vi "Translator System API.vi"(0 "Input":variant=variant("Function Name"=variant(string "Strip Path"), "Input Datatypes"=variant(string[] ["error", "int"]), "Inputs"=variant(string[] ["error in", "x"]), "Node refnum"=variant(refnum<vi> refnum), "Output Datatypes"=variant(string[] ["int"]), "Outputs"=variant(string[] ["a"])), 11 "error in (no error)":errorcluster) -> (4 "Output":variant=variant("Defines"=variant(string[] []), "Includes"=variant(string[] []), "Replaced Code"=variant(string "/* LabVIEW system function 'Strip Path' not found. */")), 15 "error out":errorcluster)   [LabVIEW 2018]
doc: "An example of how to create the Translator to convert the LabVIEW VIs to Arduino C code."
panel:
  out "Outputs":string[](array[string])
  out "Inputs":string[](array[string])
  out "Output Datatypes":string[](array[string])
  out "Input Datatypes":string[](array[string])
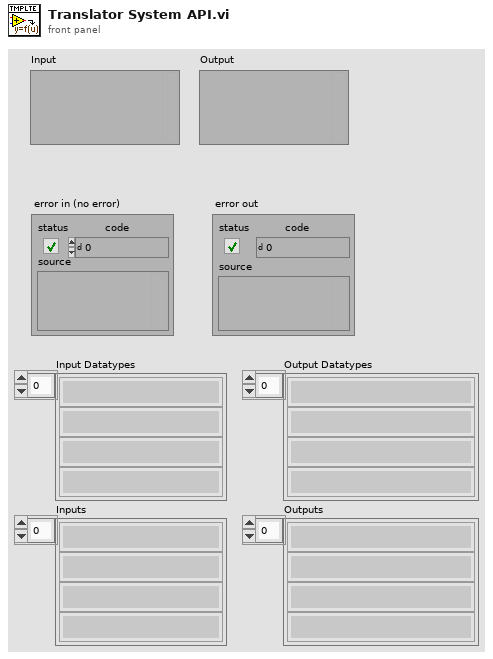
[diagram p1: front panel]
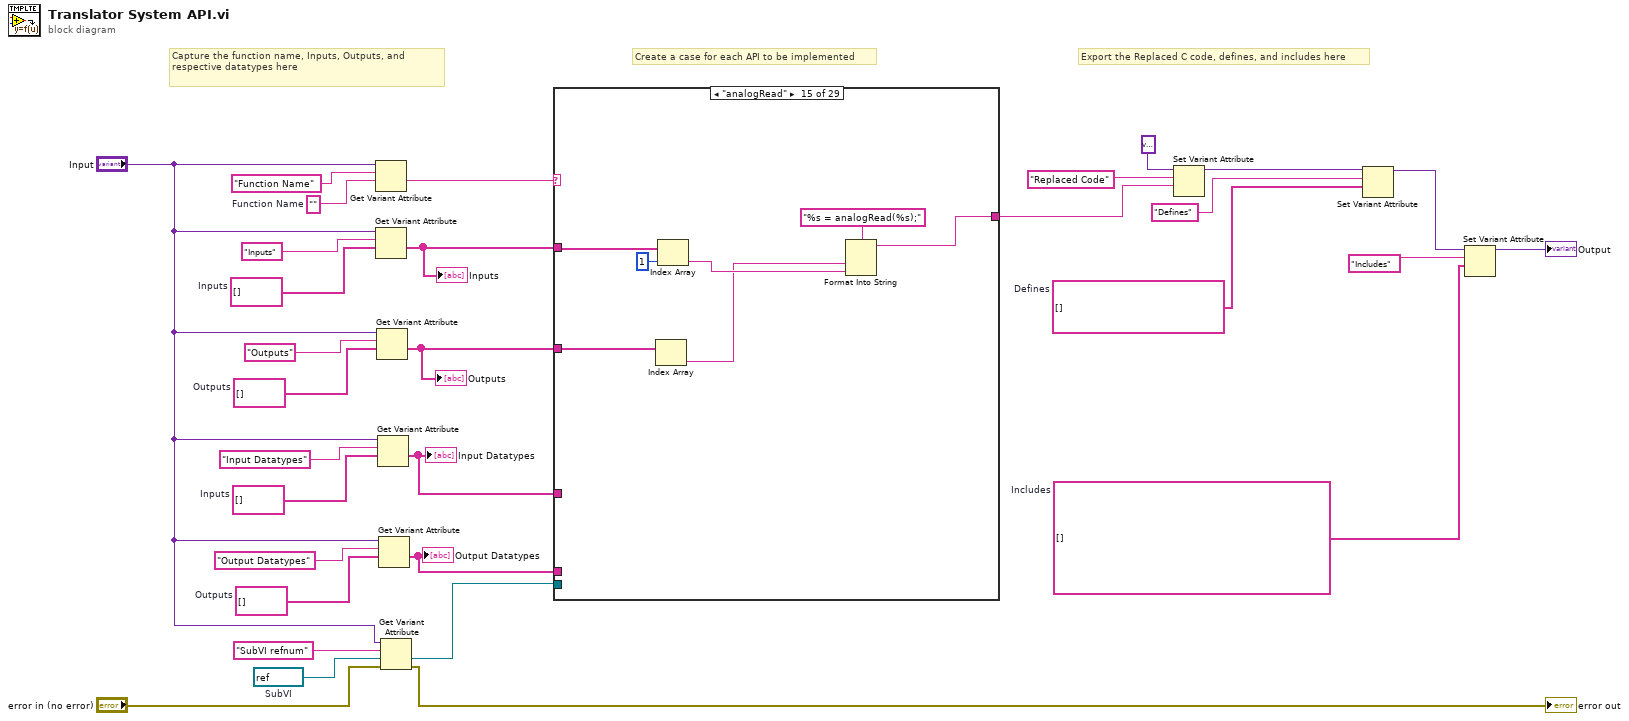
[diagram p0: block diagram]
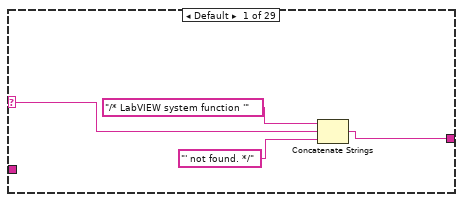
[diagram p2: hidden frame]
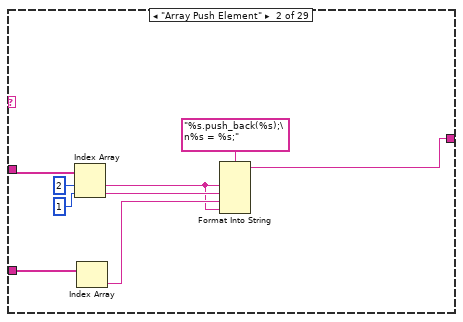
[diagram p3: hidden frame]
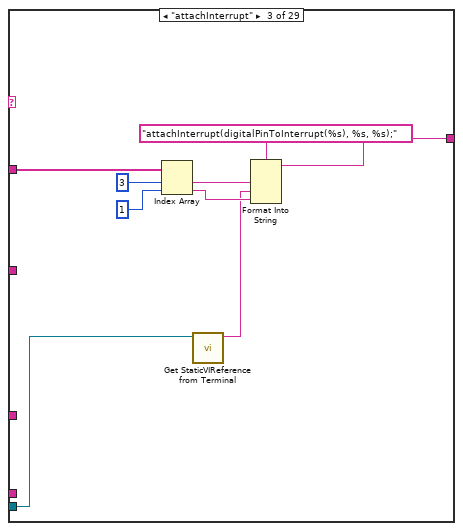
[diagram p4: hidden frame]
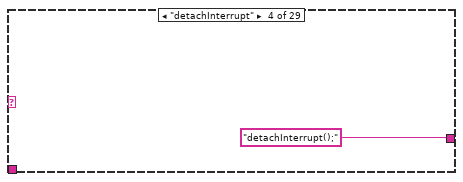
[diagram p5: hidden frame]
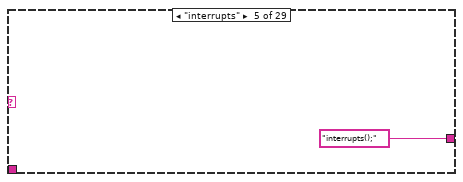
[diagram p6: hidden frame]
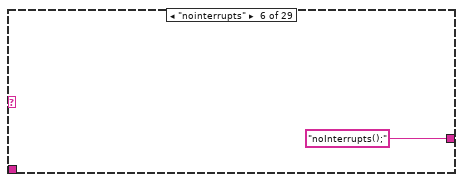
[diagram p7: hidden frame]
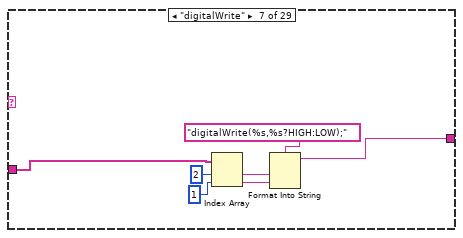
[diagram p8: hidden frame]
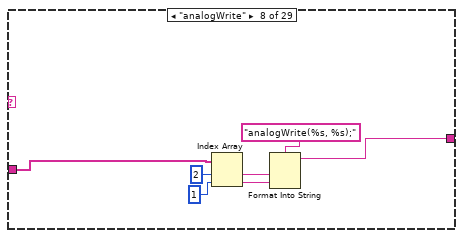
[diagram p9: hidden frame]
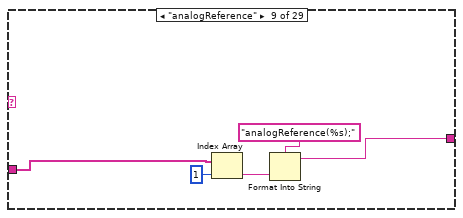
[diagram p10: hidden frame]
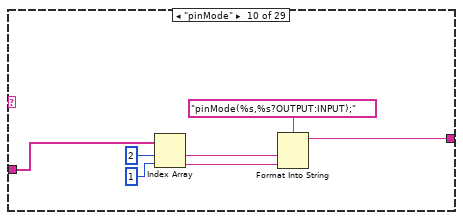
[diagram p11: hidden frame]
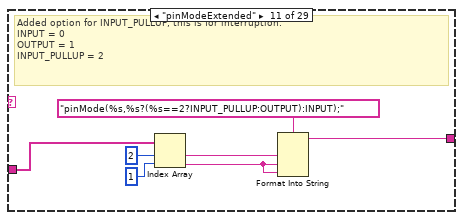
[diagram p12: hidden frame]
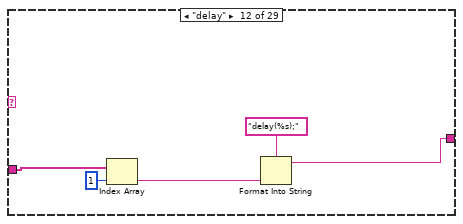
[diagram p13: hidden frame]
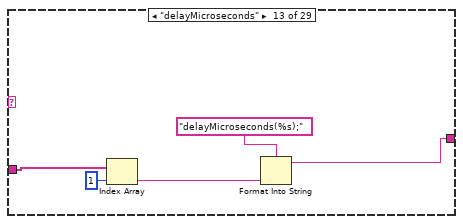
[diagram p14: hidden frame]
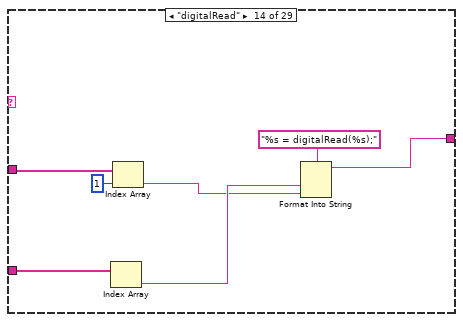
[diagram p15: hidden frame]
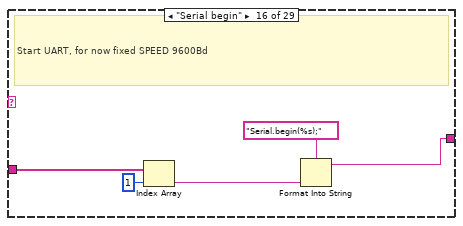
[diagram p16: hidden frame]
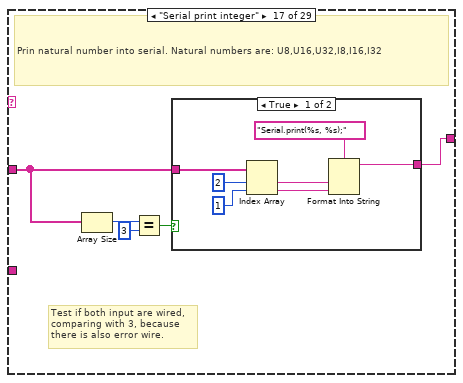
[diagram p17: hidden frame]
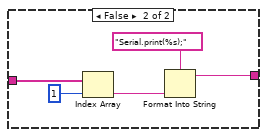
[diagram p18: hidden frame]
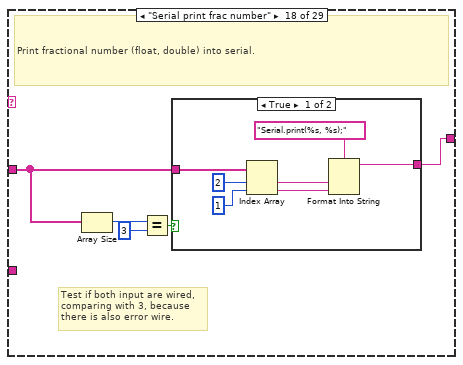
[diagram p19: hidden frame]
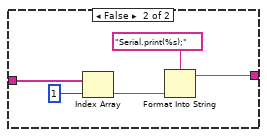
[diagram p20: hidden frame]
diagram:
  w7 = refnum<vi> refnum  # SubVI
  w4 = string[] []  # Defines
  w17 = string[] []  # Outputs
  w18 = string[] []  # Inputs
  w3 = string[] []  # Includes
  w27 = string[] []  # Outputs
  w28 = string[] []  # Inputs
  w29 = ""  # Function Name
  # "Capture the function name, Inputs, Outputs, and respective datatypes here"
  # "Export the Replaced C code, defines, and includes here"
  # "Create a case for each API to be implemented"
  n1 = Get Variant Attribute(Variant="Input", name="Function Name", default value (empty Variant)=w29) -> (value=w24:string)  [unwired: 1 in, 3 out]
  n2 = Get Variant Attribute(Variant="Input", name="Inputs", default value (empty Variant)=w28) -> (value=w14:string[])  [unwired: 1 in, 3 out]
  "Inputs" <- w14
  n3 = Get Variant Attribute(Variant="Input", name="Outputs", default value (empty Variant)=w27) -> (value=w15:string[])  [unwired: 1 in, 3 out]
  "Outputs" <- w15
  n4 = Get Variant Attribute(Variant="Input", name="Input Datatypes", default value (empty Variant)=w18) -> (value=w10:string[])  [unwired: 1 in, 3 out]
  "Input Datatypes" <- w10
  n5 = Get Variant Attribute(Variant="Input", name="Output Datatypes", default value (empty Variant)=w17) -> (value=w5:string[])  [unwired: 1 in, 3 out]
  "Output Datatypes" <- w5
  n6 = Get Variant Attribute(Variant="Input", name="SubVI refnum", default value (empty Variant)=w7, error in="error in (no error)") -> (value=w6:refnum<vi>, error out=→"error out":errorcluster)  [unwired: 2 out]
  n7 = case shown="\"analogRead\"" w24 {
    selector: w24 -> [w34 _ _ _ _ _ _ _ _ _ _ _ _ _ _ _ _ _ _ _ _ _ _ _ _ _ _ _ _]
    tunnel: [w32 w38 w49 "detachInterrupt();" ("name") "interrupts();" ("name") "noInterrupts();" ("name") w58 w65 w72 w76 w84 w90 w95 w103 w110 w115 w123 w140 w157 w158 w162 w168 w175 w192 w206 w210 "Serial.end();" ("format string") "Serial.flush();" ("format string") w215] -> w23
    tunnel: w14 -> [_ w44 w53 _ _ _ w57 w64 w71 w77 w85 w91 w96 w106 w113 w118 w120 w137 w156 _ _ w170 w171 w188 _ _ _ _ w218]
    tunnel: w15 -> [_ w39 _ _ _ _ _ _ _ _ _ _ _ w104 w111 _ _ _ _ w161 w165 _ _ _ w208 w212 _ _ _]
    tunnel: w10 -> [_ _ _ _ _ _ _ _ _ _ _ _ _ _ _ _ _ _ _ _ _ _ _ _ _ _ _ _ _]
    tunnel: w6 -> [_ _ w48 _ _ _ _ _ _ _ _ _ _ _ _ _ _ _ _ _ _ _ _ _ _ _ _ _ _]
    tunnel: w5 -> [_ _ _ _ _ _ _ _ _ _ _ _ _ _ _ _ _ _ _ _ _ _ _ _ _ _ _ _ _]
    frame Default {
      n8 = Concatenate Strings("/* LabVIEW system function '", w34, "' not found. */") -> (w32:string)
    }
    frame "Array Push Element" {
      n9 = Index Array(array=w44, index #1=2 ("index"), index #2=1 ("index")) -> (element #1=w36:string, element #2=w40:string)
      n10 = Index Array(array=w39) -> (element=w37:string)  [unwired: 1 in]
      n11 = Format Into String(format string="%s.push_back(%s);\n%s = %s;", w36, w40, w37, w36) -> (resulting string=w38:string)  [unwired: 2 in, 1 out]
    }
    frame "attachInterrupt" {
      n12 = Index Array(array=w53, index #1=3 ("index"), index #2=1 ("index")) -> (element #1=w50:string, element #2=w46:string)
      n13 = call "Get StaticVIReference from Terminal.vi"("SubVI in"=w48) -> ("String"=w45:string)  [unwired: 10 in]
      n14 = Format Into String(format string="attachInterrupt(digitalPinToInterrupt(%s), %s, %s);", w50, w45, w46) -> (resulting string=w49:string)  [unwired: 2 in, 1 out]
    }
    frame "detachInterrupt" {
    }
    frame "interrupts" {
    }
    frame "nointerrupts" {
    }
    frame "digitalWrite" {
      n15 = Index Array(array=w57, index #1=2 ("index"), index #2=1 ("index")) -> (element #1=w62:string, element #2=w61:string)
      n16 = Format Into String(format string="digitalWrite(%s,%s?HIGH:LOW);", w62, w61) -> (resulting string=w58:string)  [unwired: 2 in, 1 out]
    }
    frame "analogWrite" {
      n17 = Index Array(array=w64, index #1=2 ("index"), index #2=1 ("index")) -> (element #1=w69:string, element #2=w68:string)
      n18 = Format Into String(format string="analogWrite(%s, %s);", w69, w68) -> (resulting string=w65:string)  [unwired: 2 in, 1 out]
    }
    frame "analogReference" {
      n19 = Index Array(array=w71, index=1) -> (element=w74:string)
      n20 = Format Into String(format string="analogReference(%s);", w74) -> (resulting string=w72:string)  [unwired: 2 in, 1 out]
    }
    frame "pinMode" {
      n21 = Index Array(array=w77, index #1=2 ("index"), index #2=1 ("index")) -> (element #1=w79:string, element #2=w78:string)
      n22 = Format Into String(format string="pinMode(%s,%s?OUTPUT:INPUT);", w79, w78) -> (resulting string=w76:string)  [unwired: 2 in, 1 out]
    }
    frame "pinModeExtended" {
      # "Added option for INPUT_PULLUP, this is for interruption.\nINPUT = 0\nOUTPUT = 1\nINPUT_PULLUP = 2"
      n23 = Index Array(array=w85, index #1=2 ("index"), index #2=1 ("index")) -> (element #1=w86:string, element #2=w83:string)
      n24 = Format Into String(format string="pinMode(%s,%s?(%s==2?INPUT_PULLUP:OUTPUT):INPUT);", w86, w83, w83) -> (resulting string=w84:string)  [unwired: 2 in, 1 out]
    }
    frame "delay" {
      n25 = Index Array(array=w91, index=1) -> (element=w93:string)
      n26 = Format Into String(format string="delay(%s);", w93) -> (resulting string=w90:string)  [unwired: 2 in, 1 out]
    }
    frame "delayMicroseconds" {
      n27 = Index Array(array=w96, index=1) -> (element=w98:string)
      n28 = Format Into String(format string="delayMicroseconds(%s);", w98) -> (resulting string=w95:string)  [unwired: 2 in, 1 out]
    }
    frame "digitalRead" {
      n29 = Index Array(array=w104) -> (element=w101:string)  [unwired: 1 in]
      n30 = Index Array(array=w106, index=1) -> (element=w100:string)
      n31 = Format Into String(format string="%s = digitalRead(%s);" ("name"), w101, w100) -> (resulting string=w103:string)  [unwired: 2 in, 1 out]
    }
    frame "analogRead" {
      n32 = Index Array(array=w111) -> (element=w107:string)  [unwired: 1 in]
      n33 = Index Array(array=w113, index=1) -> (element=w108:string)
      n34 = Format Into String(format string="%s = analogRead(%s);" ("name"), w107, w108) -> (resulting string=w110:string)  [unwired: 2 in, 1 out]
    }
    frame "Serial begin" {
      # "Start UART, for now fixed SPEED 9600Bd"
      n35 = Index Array(array=w118, index=1) -> (element=w116:string)
      n36 = Format Into String(format string="Serial.begin(%s);", w116) -> (resulting string=w115:string)  [unwired: 2 in, 1 out]
    }
    frame "Serial print integer" {
      # "Test if both input are wired, comparing with 3, because there is also error wire."
      # "Prin natural number into serial. Natural numbers are: U8,U16,U32,I8,I16,I32"
      n37 = Array Size(array=w120) -> (size(s)=w122:i32)
      n38 = Equal?(x=w122, y=3) -> (x = y?=w119:bool)
      n39 = case shown="True" w119 {
        tunnel: [w130 w132] -> w123
        tunnel: w120 -> [w124 w131]
        frame True {
          n40 = Index Array(array=w124, index #1=2 ("index"), index #2=1 ("index")) -> (element #1=w126:string, element #2=w127:string)
          n41 = Format Into String(format string="Serial.print(%s, %s);", w126, w127) -> (resulting string=w130:string)  [unwired: 2 in, 1 out]
        }
        frame False {
          n42 = Index Array(array=w131, index=1) -> (element=w133:string)
          n43 = Format Into String(format string="Serial.print(%s);", w133) -> (resulting string=w132:string)  [unwired: 2 in, 1 out]
        }
      }
    }
    frame "Serial print frac number" {
      # "Test if both input are wired, comparing with 3, because there is also error wire."
      # "Print fractional number (float, double) into serial."
      n44 = Array Size(array=w137) -> (size(s)=w139:i32)
      n45 = Equal?(x=w139, y=3) -> (x = y?=w136:bool)
      n46 = case shown="True" w136 {
        tunnel: [w147 w149] -> w140
        tunnel: w137 -> [w141 w148]
        frame True {
          n47 = Index Array(array=w141, index #1=2 ("index"), index #2=1 ("index")) -> (element #1=w143:string, element #2=w144:string)
          n48 = Format Into String(format string="Serial.print(%s, %s);", w143, w144) -> (resulting string=w147:string)  [unwired: 2 in, 1 out]
        }
        frame False {
          n49 = Index Array(array=w148, index=1) -> (element=w150:string)
          n50 = Format Into String(format string="Serial.print(%s);", w150) -> (resulting string=w149:string)  [unwired: 2 in, 1 out]
        }
      }
    }
    frame "Serial print string" {
      # "Print string into serial."
      n51 = Index Array(array=w156, index=1) -> (element=w153:string)
      n52 = Format Into String(format string="Serial.print(%s);", w153) -> (resulting string=w157:string)  [unwired: 2 in, 1 out]
    }
    frame "millis" {
      # "Returns milliseconds since power on. Able to count up to 50 days."
      n53 = Index Array(array=w161) -> (element=w159:string)  [unwired: 1 in]
      n54 = Format Into String(format string="%s = millis();", w159) -> (resulting string=w158:string)  [unwired: 2 in, 1 out]
    }
    frame "micros" {
      # "eturns the number of microseconds since the Arduino board began running the current program. This number will overflow (go back to zero), after approximately 70 minutes."
      n55 = Index Array(array=w165) -> (element=w163:string)  [unwired: 1 in]
      n56 = Format Into String(format string="%s = micros();", w163) -> (resulting string=w162:string)  [unwired: 2 in, 1 out]
    }
    frame "Serial println string" {
      # "Print string into UART."
      n57 = Index Array(array=w170, index=1) -> (element=w169:string)
      n58 = Format Into String(format string="Serial.println(%s);", w169) -> (resulting string=w168:string)  [unwired: 2 in, 1 out]
    }
    frame "Serial println integer" {
      # "Test if both input are wired, comparing with 3, because there is also error wire."
      # "Print natural number into UART (short, byte, int), with specified base (hexadecimal, octal, decadic, binary)"
      n59 = Array Size(array=w171) -> (size(s)=w174:i32)
      n60 = Equal?(x=w174, y=3) -> (x = y?=w173:bool)
      n61 = case shown="True" w173 {
        tunnel: w171 -> [w176 w184]
        tunnel: [w177 w181] -> w175
        frame False {
          n62 = Index Array(array=w176, index=1) -> (element=w180:string)
          n63 = Format Into String(format string="Serial.println(%s);", w180) -> (resulting string=w177:string)  [unwired: 2 in, 1 out]
        }
        frame True {
          n64 = Index Array(array=w184, index #1=2 ("index"), index #2=1 ("index")) -> (element #1=w187:string, element #2=w182:string)
          n65 = Format Into String(format string="Serial.println(%s, %s);", w187, w182) -> (resulting string=w181:string)  [unwired: 2 in, 1 out]
        }
      }
    }
    frame "Serial println frac number" {
      # "Test if both input are wired, comparing with 3, because there is also error wire."
      # "Print fractional number into UART, user can specify precision, so there is case if preciosion wired or not."
      n66 = Array Size(array=w188) -> (size(s)=w191:i32)
      n67 = Equal?(x=w191, y=3) -> (x = y?=w190:bool)
      n68 = case shown="True" w190 {
        tunnel: w188 -> [w193 w201]
        tunnel: [w194 w198] -> w192
        frame False {
          n69 = Index Array(array=w193, index=1) -> (element=w197:string)
          n70 = Format Into String(format string="Serial.println(%s);", w197) -> (resulting string=w194:string)  [unwired: 2 in, 1 out]
        }
        frame True {
          n71 = Index Array(array=w201, index #1=2 ("index"), index #2=1 ("index")) -> (element #1=w204:string, element #2=w199:string)
          n72 = Format Into String(format string="Serial.println(%s, %s);", w204, w199) -> (resulting string=w198:string)  [unwired: 2 in, 1 out]
        }
      }
    }
    frame "Serial read" {
      n73 = Index Array(array=w208) -> (element=w205:string)  [unwired: 1 in]
      n74 = Format Into String(format string="%s = Serial.read();", w205) -> (resulting string=w206:string)  [unwired: 2 in, 1 out]
    }
    frame "Serial available" {
      n75 = Index Array(array=w212) -> (element=w209:string)  [unwired: 1 in]
      n76 = Format Into String(format string="%s = Serial.available();", w209) -> (resulting string=w210:string)  [unwired: 2 in, 1 out]
    }
    frame "Serial end" {
    }
    frame "Serial flush" {
    }
    frame "Serial write" {
      n77 = Index Array(array=w218, index=1) -> (element=w216:string)
      n78 = Format Into String(format string="Serial.write(%s);", w216) -> (resulting string=w215:string)  [unwired: 2 in, 1 out]
    }
  }
  n79 = Set Variant Attribute(Variant=variant ("variant"), name="Replaced Code", value=w23) -> (Variant out=w13:variant)  [unwired: 1 in, 2 out]
  n80 = Set Variant Attribute(Variant=w13, name="Defines", value=w4) -> (Variant out=w12:variant)  [unwired: 1 in, 2 out]
  n81 = Set Variant Attribute(Variant=w12, name="Includes", value=w3) -> (Variant out=→"Output":variant)  [unwired: 1 in, 2 out]
